vi "UploadScript.vi"(8 "error in":errorcluster, 10 "Script File":path=path "sample.script.py", 11 "Comport":refnum<visa-resource-name>="COM8") -> (0 "error out":errorcluster, 1 "DownloadSuccessful":bool, 2 "Reply":string, 3 "Comport Out":refnum<visa-resource-name>)   [LabVIEW 2020, in "MicroPython.lvlib"]
doc: "Upload a script (*.py) to the target device running micropython"
uses:
  MicroPython.lvlib
  <vilib>/regexp/Match Regular Expression.xnode
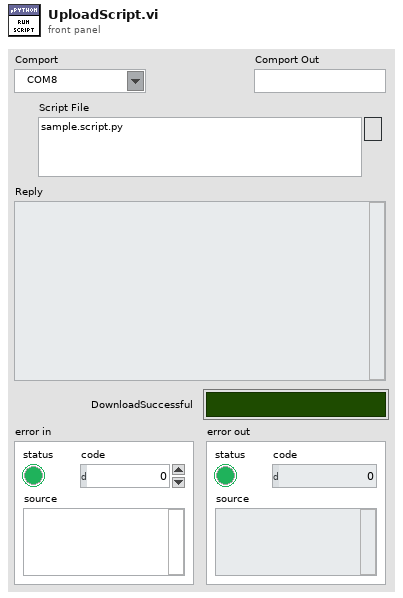
[diagram p1: front panel]
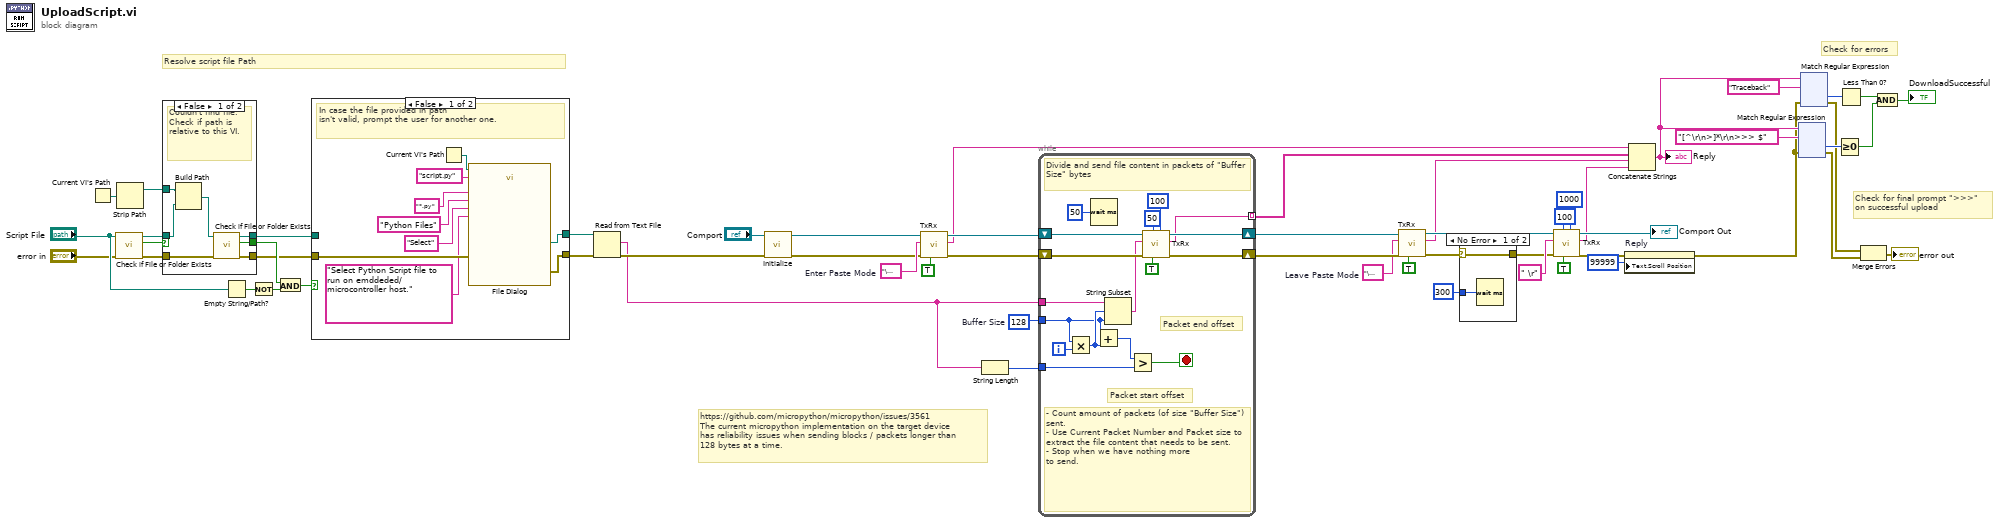
[diagram p0: block diagram]
diagram:
  w16 = 128  # Buffer Size
  w38 = "\u0004"  # Leave Paste Mode
  w40 = "\u0005"  # Enter Paste Mode
  # "Check for final prompt \">>>\"\non successful upload"
  # "Check for errors"
  # "https://github.com/micropython/micropython/issues/3561\nThe current micropython implementation on the target device\nhas reliability issues when sending blocks / packets longer than\n128 bytes at a time."
  # "Resolve script file Path"
  n1 = Current VI's Path() -> (path=w55:path)
  n2 = call <vilib>:"Check if File or Folder Exists.vi"("error in (no error)"="error in", "path"="Script File") -> ("error out"=w50:errorcluster, "file or folder exists?"=w53:bool, "dup path"=w52:path)  [unwired: 7 in]
  n3 = Strip Path(path=w55) -> (stripped path=w56:path)  [unwired: 1 out]
  n4 = case shown="False" w53 {
    selector: w53 -> [_ w65]
    tunnel: [w62 w67] -> w49
    tunnel: w50 -> [w64 w67]
    tunnel: [w63 w66] -> w51
    tunnel: w52 -> [w59 w66]
    tunnel: [w61 w65] -> w54
    tunnel: w56 -> [w58 _]
    frame False {
      # "Couldn't find file.\nCheck if path is relative to this VI."
      n5 = Build Path(base path=w58, name or relative path=w59) -> (appended path=w60:path)
      n6 = call <vilib>:"Check if File or Folder Exists.vi"("error in (no error)"=w64, "path"=w60) -> ("error out"=w62:errorcluster, "file or folder exists?"=w61:bool, "dup path"=w63:path)  [unwired: 7 in]
    }
    frame True {
      # "Found file,\nNo worries"
    }
  }
  n7 = Empty String/Path?(string/path="Script File") -> (empty?=w47:bool)
  n8 = Not(x=w47) -> (.not. x?=w48:bool)
  n9 = And(x=w54, y=w48) -> (x .and. y?=w46:bool)
  n10 = case shown="False" w46 {
    tunnel: w51 -> [_ w78]
    tunnel: [w76 w78] -> w42
    tunnel: w49 -> [w74 w77]
    tunnel: [w75 w77] -> w43
    frame False {
      # "In case the file provided in path\nisn't valid, prompt the user for another one."
      n11 = Current VI's Path() -> (path=w73:path)
      n12 = call "File Dialog"("start path"=w73, "prompt"="Select Python Script file to run on emddeded/microcontroller host.", "button label"="Select", "default name"="script.py", "error in"=w74, "pattern (all files)"="*.py", "pattern label"="Python Files") -> ("selected path"=w76:path, "error out"=w75:errorcluster)  [unwired: 5 in, 2 out]
    }
    frame True {
      # "We have a valid file. No worries"
    }
  }
  n13 = Read from Text File(file (use dialog)=w42, error in=w43) -> (text=w15:string, error out=w18:errorcluster)  [unwired: 2 in, 2 out]
  n14 = call "Initialize.vi"("error in"=w18, "Comport"="Comport") -> ("error out"=w17:errorcluster, "Comport Out"=w19:refnum<visa-resource-name>)  [unwired: 8 in]
  n15 = call "TxRx.vi"("Receive?"=TRUE, "error in"=w17, "Tx Message"=w40, "VISA Resource Name In"=w19) -> ("error out"=w34:errorcluster, "Rx Message"=w29:string, "VISA Resource Name Out"=w39:refnum<visa-resource-name>)  [unwired: 5 in]
  n16 = String Length(string=w15) -> (length=w14:i32)
  n17 = while {
    shift-right: [w93] -> w37
    shift-left: w39 -> [w94]
    shift-right: [w95] -> w57
    shift-left: w34 -> [w92]
    tunnel: w15 -> [w90]
    tunnel: w16 -> [w86]
    tunnel: w14 -> [w84]
    tunnel: [w82] -> w1 mode=indexing
    i -> [w89]
    stop <- w83 stop-if-true
    # "Packet end offset"
    # "Packet start offset"
    # "- Count amount of packets (of size \"Buffer Size\") sent.\n- Use Current Packet Number and Packet size to extract the file content that needs to be sent.\n- Stop when we have nothing more\nto send."
    # "Divide and send file content in packets of \"Buffer Size\" bytes"
    n18 = Multiply(x=w86, y=w89) -> (x*y=w87:i32)
    n19 = Wait (ms)(milliseconds to wait=u32 50) -> ()  [unwired: 1 out]
    n20 = Add(x=w86, y=w87) -> (x+y=w85:i32)
    n21 = String Subset(string=w90, offset (0)=w87, length (rest)=w86) -> (substring=w88:string)
    n22 = Greater?(x=w85, y=w84) -> (0:w83:bool)
    n23 = call "TxRx.vi"("Timeout (Ms)"=u32 100 ("ms Timeout"), "Receive?"=TRUE, "Wait Before Read (Ms)"=u32 50 ("ms Wait Before Read"), "error in"=w92, "Tx Message"=w88, "VISA Resource Name In"=w94) -> ("error out"=w95:errorcluster, "Rx Message"=w82:string, "VISA Resource Name Out"=w93:refnum<visa-resource-name>)  [unwired: 3 in]
  }
  n24 = call "TxRx.vi"("Receive?"=TRUE, "error in"=w57, "Tx Message"=w38, "VISA Resource Name In"=w37) -> ("error out"=w25:errorcluster, "Rx Message"=w28:string, "VISA Resource Name Out"=w32:refnum<visa-resource-name>)  [unwired: 5 in]
  n25 = case shown="No Error" w25 {
    selector: w25 -> [w96 w98]
    tunnel: u32 300 ("milliseconds to wait") -> [w97 _]
    tunnel: [w96 w98] -> w24
    frame No Error {
      n26 = Wait (ms)(milliseconds to wait=w97) -> ()  [unwired: 1 out]
    }
    frame Error {
    }
  }
  n27 = call "TxRx.vi"("Timeout (Ms)"=u32 1000 ("ms Timeout"), "Receive?"=TRUE, "Wait Before Read (Ms)"=u32 100 ("ms Wait Before Read"), "error in"=w24, "Tx Message"=" \r", "VISA Resource Name In"=w32) -> ("error out"=w23:errorcluster, "Rx Message"=w27:string, "VISA Resource Name Out"=→"Comport Out":refnum<visa-resource-name>)  [unwired: 3 in]
  n28 = property on="Reply" class="Str"(error in=w23, "Text.Scroll Position"=u32 99999) -> (error out=w5:errorcluster)  [unwired: 1 in, 1 out]
  n29 = Concatenate Strings(w29, w1, w28, w27) -> (w11:string)
  "Reply" <- w11
  n30 = xnode "Match Regular Expression"("input string"=w11, "regular expression"="[^\r\n>]*\r\n>>> $", "error in"=w5) -> ("offset past match"=w21:i32, "error out"=w2:errorcluster)  [unwired: 3 in, 3 out]
  n31 = xnode "Match Regular Expression"("input string"=w11, "regular expression"="Traceback", "error in"=w5) -> ("offset past match"=w9:i32, "error out"=w3:errorcluster)  [unwired: 3 in, 3 out]
  n32 = Greater Or Equal To 0?(x=w21) -> (x >= 0?=w7:bool)
  n33 = Less Than 0?(x=w9) -> (x < 0?=w8:bool)
  n34 = Merge Errors(w3, w2) -> (→"error out":errorcluster)
  n35 = And(x=w8, y=w7) -> (x .and. y?=→"DownloadSuccessful":bool)
